vi "PH_USB600x_AnalogReader.acquire waveform data.vi"(0 "i ref in":refnum<vi>, 3 "Device Timeout [sec] (1)":dbl=1.0, 5 "error in (no error)":errorcluster) -> (14 "i ref out":refnum<vi>, 19 "error out":errorcluster)   [LabVIEW 2014, in "PH_USB600x_AnalogReader.lvlib"]
doc: "Acquires the waveform from the device.\n\nLicense Agreement for the BaseProcess class:\n\nCopyright (C)\nGesellschaft für Schwerionenforschung, GSI\nPlanckstr. 1\n64291 Darmstadt\nGermany\n\nContact: D.Beck@gsi.de \n\nThis program is free software; you can redistribute it and/or modify it under the terms of the \nGNU General Public License as published by the Free Software Foundation; either version 2 of the license, or (at your option) any later version.\n\nThis program is distributed in the hope that it will be useful, but WITHOUT ANY WARRANTY; without even the implied warranty of MERCHANTABILITY or FITNESS FOR A PARTICULAR PURPOSE. See the GNU General License for more details (http://www.gnu.org).\n\nGesellschaft für Schwerionenforschung, GSI\nPlanckstr. 1, 64291 Darmstadt, Germany\nFor all questions and ideas contact: M.Richter@gsi.de, H.Brand@gsi.de or D.Beck@gsi.de.\nLast update: 25-SEP-2002"
uses:
  PH_USB600x_AnalogReader.lvlib
  PH_StatusHandler/PH_StatusHandler.Status.ctl
  <vilib>/DAQmx/read.llb/DAQmx Read (Analog Wfm 1Chan NSamp).vi
  <vilib>/DAQmx/read.llb/DAQmx Read (Analog Wfm 1Chan 1Samp).vi
  PH_StatusHandler/PH_StatusHandler.lvlib
  PH_Common/PH_Common.lvlib
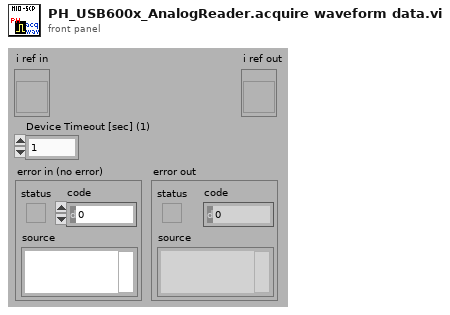
[diagram p1: front panel]
types:
  T1 = typedef "PH_USB600x_AnalogReader.lvlib/PH_USB600x_AnalogReader.i attribute.ctl" = cluster{"GUI Refs":cluster{"Delete":refnum<vi>, "Status":refnum<vi>, "Timeout":refnum<vi>, "Acquire Waveform":refnum<vi>, "Timing":refnum<vi>, "Graph":refnum<vi>, "Prdc Interval":refnum<vi>, "Formula":refnum<vi>}, "Device Settings":cluster{"AIChannel":refnum<k21>, "channelName":string, "Status":T2}, "Timing":T3, "Prdc Interval":dbl, "Lin Scaling":T4, "Data":cluster{"t0":timestamp, dbl}[]}
  T2 = typedef "PH_StatusHandler.lvlib/PH_StatusHandler.Status.ctl" = i16
  T3 = typedef "PH_USB600x_AnalogReader.lvlib/PH_USB600x_AnalogReader.Timing.ctl" = cluster{"Samples per Channel":i32, "Rate":dbl}
  T4 = typedef "PH_USB600x_AnalogReader.lvlib/PH_USB600x_AnalogReader.Lin Scaling.ctl" = cluster{"Slope [Unit/V]":dbl, "Offset [Unit]":dbl, "Y-Unit":string, "Y-Label":string}
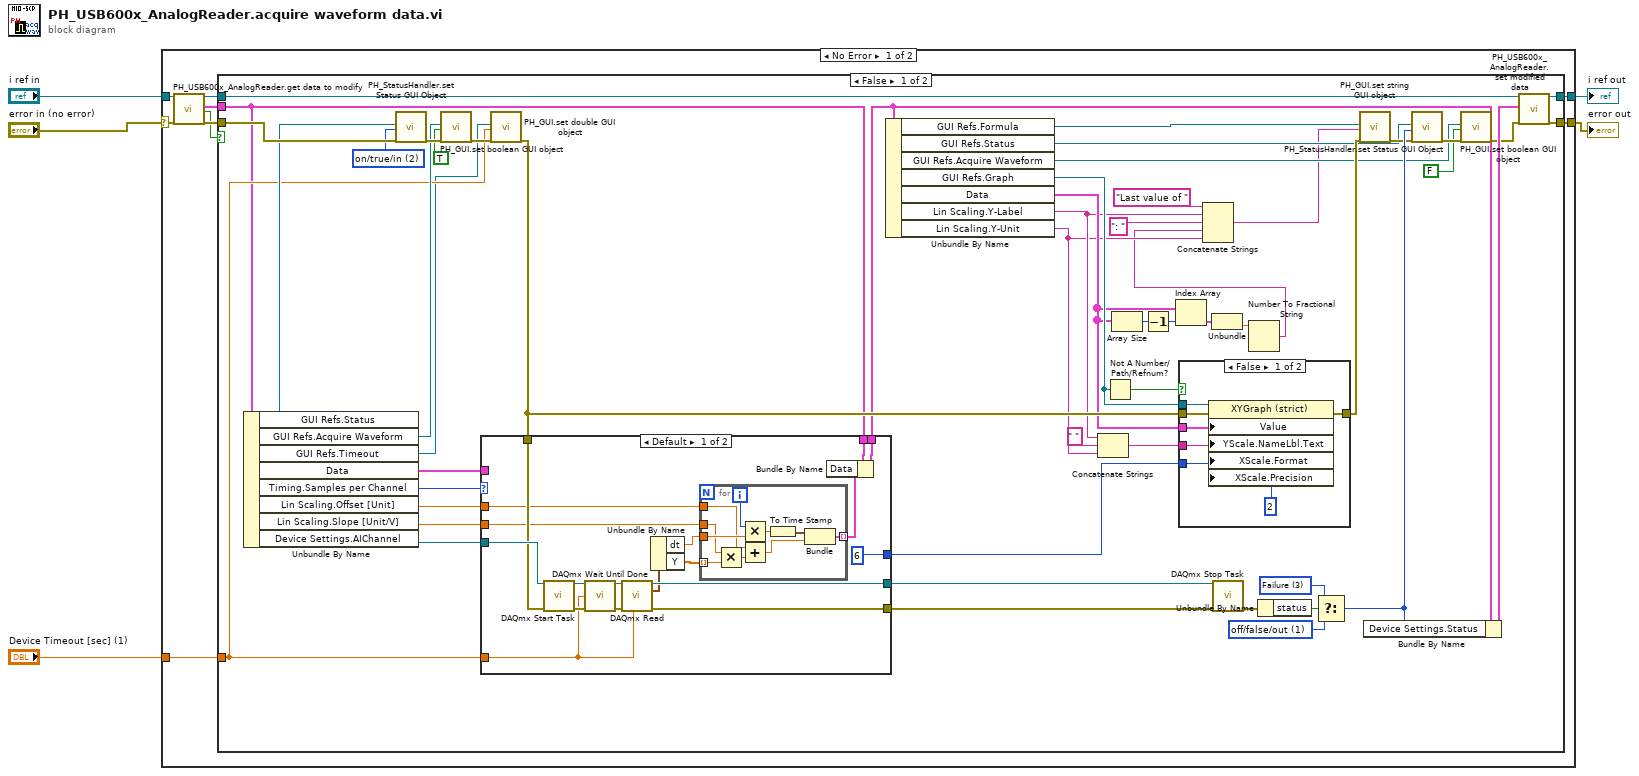
[diagram p0: block diagram]
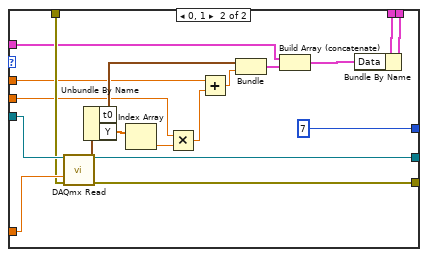
[diagram p3: hidden frame]
diagram:
  n1 = case shown="No Error" "error in (no error)" {
    selector: "error in (no error)" -> [w12 w124]
    tunnel: "i ref in" -> [w14 w125]
    tunnel: [w8 w125] -> w4
    tunnel: "Device Timeout [sec] (1)" -> [w10 _]
    tunnel: [w7 w124] -> w2
    frame No Error {
      n2 = call "PH_USB600x_AnalogReader.get data to modify.vi"("i ref in"=w14, "error in (no error)"=w12) -> ("i ref out"=w9:refnum<vi>, "i attribute"=w13:T1, "timed out"=w6:bool, "error out"=w11:errorcluster)  [unwired: 14 in]
      n3 = case shown="False" w6 {
        tunnel: w13 -> [w25 _]
        tunnel: w11 -> [w54 w122]
        tunnel: w10 -> [w28 _]
        tunnel: w9 -> [w64 w123]
        tunnel: [w63 w123] -> w8
        tunnel: [w62 w122] -> w7
        frame False {
          w53 = T2 2 items=["no info", "off/false/out", "on/true/in", "Failure", "Alarm", "Status 1", "Status 2", "Status 3"] ("Device Settings.Status")
          w57 = T2 1 items=["no info", "off/false/out", "on/true/in", "Failure", "Alarm", "Status 1", "Status 2", "Status 3"] ("Device Settings.Status")
          w58 = T2 3 items=["no info", "off/false/out", "on/true/in", "Failure", "Alarm", "Status 1", "Status 2", "Status 3"] ("Device Settings.Status")
          n4 = Unbundle By Name(w25) -> ("GUI Refs.Status"=w36:refnum<vi>, "GUI Refs.Acquire Waveform"=w34:refnum<vi>, "GUI Refs.Timeout"=w26:refnum<vi>, "Data"=w31:cluster{"t0":timestamp, dbl}[], "Timing.Samples per Channel"=w60:i32, "Lin Scaling.Offset [Unit]"=w29:dbl, "Lin Scaling.Slope [Unit/V]"=w30:dbl, "Device Settings.AIChannel"=w45:refnum<k21>)
          n5 = call "PH_StatusHandler.set Status GUI Object.vi"("PH Status Ref"=w36, "Value"=w53, "error in (no error)"=w54) -> ("error out"=w51:errorcluster)  [unwired: 16 in]
          n6 = call "PH_GUI.set boolean GUI object.vi"("Boolean Knob GUI Ref"=w34, "Value"=TRUE, "error in (no error)"=w51) -> ("error out"=w46:errorcluster)  [unwired: 16 in]
          n7 = call "PH_GUI.set double GUI object.vi"("GUI object Ref"=w26, "value"=w28, "error in (no error)"=w46) -> ("error out"=w27:errorcluster)  [unwired: 16 in]
          n8 = case shown="Default" w60 {
            tunnel: [w92 w121] -> w66
            tunnel: w45 -> [w90 w120]
            tunnel: [w91 w119] -> w65
            tunnel: w28 -> [w85 w118]
            tunnel: w27 -> [w81 w109]
            tunnel: [u8 6 ("X Scale.Format & Precision:Format") u8 7 ("X Scale.Format & Precision:Format")] -> w44
            tunnel: w31 -> [_ w108]
            tunnel: w30 -> [w79 w107]
            tunnel: w29 -> [w78 w106]
            tunnel: w25 -> [w76 w104]
            tunnel: [w77 w103] -> w24
            frame Default {
              n9 = call <vilib>:"DAQmx Start Task.vi"("task/channels in"=w90, "error in"=w81) -> ("task out"=w89:refnum<k21>, "error out"=w87:errorcluster)  [unwired: 12 in]
              n10 = call <vilib>:"DAQmx Wait Until Done.vi"("task/channels in"=w89, "timeout (sec)"=w85, "error in"=w87) -> ("task out"=w88:refnum<k21>, "error out"=w86:errorcluster)  [unwired: 11 in]
              n11 = call-poly <vilib>:"DAQmx Read.vi"("task/channels in"=w88, "timeout"=w85, "error in"=w86) -> ("task out"=w92:refnum<k21>, "data"=w82:waveform(dbl), "error out"=w91:errorcluster)  [unwired: 10 in]
              n12 = Unbundle By Name(w82) -> ("dt"=w83:dbl, "Y"=w84:dbl[])
              n13 = for {
                tunnel: w84 -> [w96] mode=indexing
                tunnel: [w102] -> w75 mode=indexing
                tunnel: w83 -> [w101]
                tunnel: w78 -> [w94]
                tunnel: w79 -> [w93]
                i -> [w100]
                n14 = Multiply(x=w93, y=w96) -> (x*y=w97:dbl)
                n15 = Multiply(x=w100, y=w101) -> (x*y=w99:dbl)
                n16 = Add(x=w94, y=w97) -> (x+y=w95:dbl)
                n17 = To Time Stamp(1:w99) -> (0:w98:timestamp)
                n18 = Bundle(w98, w95) -> (w102:cluster{timestamp, dbl})  [unwired: 1 in]
              }
              n19 = Bundle By Name(cluster=w76, "Data"=w75) -> (w77:T1)
            }
            frame 0, 1 {
              n20 = call-poly <vilib>:"DAQmx Read.vi"("task/channels in"=w120, "timeout"=w118, "error in"=w109) -> ("task out"=w121:refnum<k21>, "data"=w117:waveform(dbl), "error out"=w119:errorcluster)  [unwired: 10 in]
              n21 = Unbundle By Name(w117) -> ("t0"=w113:timestamp, "Y"=w116:dbl[])
              n22 = Index Array(array=w116) -> (element=w111:dbl)  [unwired: 1 in]
              n23 = Multiply(x=w107, y=w111) -> (x*y=w112:dbl)
              n24 = Add(x=w106, y=w112) -> (x+y=w110:dbl)
              n25 = Bundle("t0"=w113, w110) -> (w115:cluster{"t0":timestamp, dbl})  [unwired: 1 in]
              n26 = Build Array (concatenate)(w108, w115) -> (w105:cluster{"t0":timestamp, dbl}[])
              n27 = Bundle By Name(cluster=w104, "Data"=w105) -> (w103:T1)
            }
          }
          n28 = Unbundle By Name(w24) -> ("GUI Refs.Formula"=w37:refnum<vi>, "GUI Refs.Status"=w35:refnum<vi>, "GUI Refs.Acquire Waveform"=w33:refnum<vi>, "GUI Refs.Graph"=w32:refnum<vi>, "Data"=w23:cluster{"t0":timestamp, dbl}[], "Lin Scaling.Y-Label"=w19:string, "Lin Scaling.Y-Unit"=w17:string)
          n29 = Concatenate Strings(w19, " " ("string"), w17) -> (w21:string)
          n30 = Not A Number/Path/Refnum?(number/path/refnum=w32) -> (NaN/Path/Refnum?=w52:bool)
          n31 = Array Size(array=w23) -> (size(s)=w41:i32)
          n32 = Decrement(x=w41) -> (x-1=w40:i32)
          n33 = Index Array(array=w23, index=w40) -> (element=w39:cluster{"t0":timestamp, dbl})
          n34 = case shown="False" w52 {
            tunnel: w32 -> [w73 _]
            tunnel: w27 -> [w72 w74]
            tunnel: [w71 w74] -> w42
            tunnel: w23 -> [w69 _]
            tunnel: w44 -> [w70 _]
            tunnel: w21 -> [w67 _]
            frame False {
              n35 = property class="XYGraph (strict)"(reference=w73, error in=w72, "Value"=w69, "YScale.NameLbl.Text"=w67, "XScale.Format"=w70, "XScale.Precision"=u8 2 ("X Scale.Format & Precision:Format")) -> (error out=w71:errorcluster)  [unwired: 1 out]
            }
            frame True {
            }
          }
          n36 = Unbundle(w39) -> (w38:dbl)  [unwired: 1 out]
          n37 = call <vilib>:"DAQmx Stop Task.vi"("task/channels in"=w66, "error in"=w65) -> ("error out"=w56:errorcluster)  [unwired: 12 in, 1 out]
          n38 = Number To Fractional String(number=w38) -> (F-format string=w15:string)  [unwired: 3 in]
          n39 = Concatenate Strings("Last value of " ("string"), w19, ": " ("string"), w15, w17) -> (w16:string)
          n40 = Unbundle By Name(w56) -> ("status"=w59:bool)
          n41 = Select(t=w58, s=w59, f=w57) -> (s? t:f=w55:T2)
          n42 = call "PH_GUI.set string GUI object.vi"("GUI object Ref"=w37, "Text"=w16, "error in"=w42) -> ("error out"=w43:errorcluster)  [unwired: 16 in]
          n43 = Bundle By Name(cluster=w24, "Device Settings.Status"=w55) -> (w61:T1)
          n44 = call "PH_StatusHandler.set Status GUI Object.vi"("PH Status Ref"=w35, "Value"=w55, "error in (no error)"=w43) -> ("error out"=w49:errorcluster)  [unwired: 16 in]
          n45 = call "PH_GUI.set boolean GUI object.vi"("Boolean Knob GUI Ref"=w33, "Value"=FALSE, "error in (no error)"=w49) -> ("error out"=w48:errorcluster)  [unwired: 16 in]
          n46 = call "PH_USB600x_AnalogReader.set modified data.vi"("i ref in"=w64, "i attribute"=w61, "error in (no error)"=w48) -> ("i ref out"=w63:refnum<vi>, "error out"=w62:errorcluster)  [unwired: 15 in]
        }
        frame True {
        }
      }
    }
    frame Error {
    }
  }
  "error out" <- w2
  "i ref out" <- w4
